vi "NIDCPower_channel_ganging - configure voltage limit.vi"(7 "Limit Symmetry":i32(ring)=1 items=["Symmetric", "Asymmetric"], 8 "error in (no error)":errorcluster, 9 "voltage limit/hi":dbl format="%#.6p", 10 "voltage limit lo":dbl format="%#.6p", 11 "Ganged Session In":T1={"Ganged Config"=enum."Parallel", "Session List"=[], "Session Mode"=[], "Channel"=[]}) -> (0 "error out":errorcluster, 3 "Ganged Session Out":T1)   [LabVIEW 2021]
uses:
  ctl/NIDCPower_channel_ganging - ctl - ganged session.ctl
  ctl/NIDCPower_channel_ganging - ctl - ganged config.ctl
  ctl/NIDCPower_channel_ganging - ctl - channel mode.ctl
panel:
  in  "Channel":string="0"
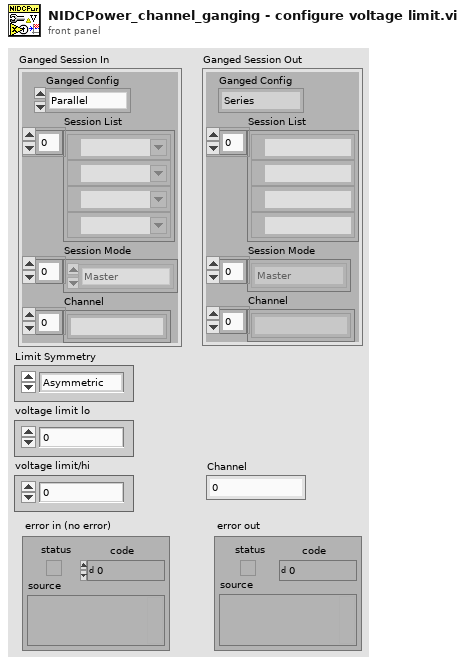
[diagram p1: front panel]
types:
  T1 = typedef "NIDCPower_channel_ganging - ctl - ganged session.ctl" = cluster{"Ganged Config":T2, "Session List":refnum<k15>[], "Session Mode":T3[], "Channel":string[]}
  T2 = typedef "NIDCPower_channel_ganging - ctl - ganged config.ctl" = enum32{"Series", "Parallel", "Manual"}
  T3 = typedef "NIDCPower_channel_ganging - ctl - channel mode.ctl" = enum32{"Master", "Slave", "Slave - Inverted"}
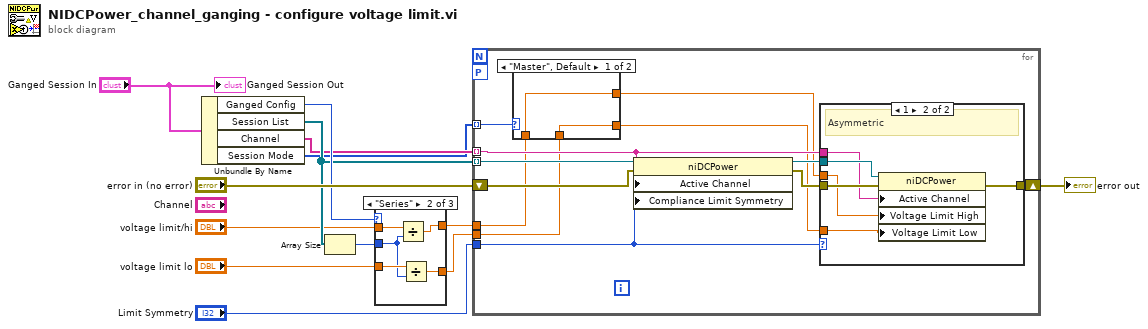
[diagram p0: block diagram]
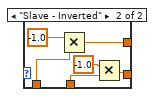
[diagram p4: hidden frame]
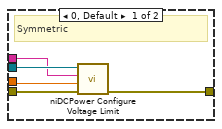
[diagram p5: hidden frame]
diagram:
  n1 = Unbundle By Name("Ganged Session In") -> ("Ganged Config"=w11:T2, "Session List"=w9:refnum<k15>[], "Channel"=w2:string[], "Session Mode"=w1:T3[])
  n2 = Array Size(array=w9) -> (size(s)=w7:i32)
  n3 = case shown="\"Series\"" w11 {
    tunnel: w7 -> [_ w16 _]
    tunnel: "voltage limit/hi" -> [w15 w20 w22]
    tunnel: [w15 w19 w22] -> w8
    tunnel: "voltage limit lo" -> [w14 w18 w21]
    tunnel: [w14 w17 w21] -> w3
    frame "Parallel" {
    }
    frame "Series" {
      n4 = Divide(x=w20, y=w16) -> (x/y=w19:dbl)
      n5 = Divide(x=w18, y=w16) -> (x/y=w17:dbl)
    }
    frame "Manual" {
    }
  }
  n6 = for {
    shift-right: [w34] -> w12
    shift-left: "error in (no error)" -> [w30]
    tunnel: w9 -> [w33] mode=indexing
    tunnel: w8 -> [w26]
    workers-P: _ -> [_]
    tunnel: "Limit Symmetry" -> [w29]
    tunnel: w3 -> [w25]
    tunnel: w2 -> [w28] mode=indexing
    tunnel: w1 -> [w27] mode=indexing
    n7 = case shown="\"Master\", Default" w27 {
      tunnel: w26 -> [w36 w40]
      tunnel: w25 -> [w35 w39]
      tunnel: [w36 w38] -> w24
      tunnel: [w35 w37] -> w23
      frame "Master", Default {
      }
      frame "Slave - Inverted" {
        n8 = Multiply(x=-1.0, y=w40) -> (x*y=w38:dbl)
        n9 = Multiply(x=-1.0, y=w39) -> (x*y=w37:dbl)
      }
    }
    n10 = property class="niDCPower"(reference=w33, error in=w30, "Active Channel"=w28, "Compliance Limit Symmetry"=w29) -> (reference out=w32:refnum<k15>, error out=w31:errorcluster)
    n11 = case shown="1" w29 {
      tunnel: w31 -> [w47 w51]
      tunnel: w32 -> [w46 w52]
      tunnel: [w45 w53] -> w34
      tunnel: w28 -> [w44 w50]
      tunnel: w24 -> [w43 w49]
      tunnel: w23 -> [_ w48]
      frame 0, Default {
        # "Symmetric"
        n12 = call <instrlib>:"niDCPower Configure Voltage Limit.vi"("error in (no error)"=w47, "voltage limit"=w43, "channel name"=w44, "instrument handle"=w46) -> ("error out"=w45:errorcluster)  [unwired: 6 in, 1 out]
      }
      frame 1 {
        # "Asymmetric"
        n13 = property class="niDCPower"(reference=w52, error in=w51, "Active Channel"=w50, "Voltage Limit High"=w49, "Voltage Limit Low"=w48) -> (error out=w53:errorcluster)  [unwired: 1 out]
      }
    }
  }
  "error out" <- w12
  "Ganged Session Out" <- "Ganged Session In"
